vi "Control Panel.vi"(8 "error in (no error)":errorcluster, 11 "Magna Power in":refnum<class "Magna Power.lvclass">) -> (0 "error out":errorcluster, 3 "Magna Power out":refnum<class "Magna Power.lvclass">)   [LabVIEW 2017, in "Magna Power.lvclass"]
doc: "(Dynamic) A user-level application that simulates the physical front panel of the Instrument. Provide the user with buttons to manually control features of the instrument, and provide indicators of its current state."
uses:
  Magna Power.lvclass
  Magna Power.lvclass/Magna Power.ctl
panel:
  in  "Reset Power Supply":bool
  in  "Zero field":bool
  out "Actual Voltage (V)":dbl
  out "Actual Current (A)":dbl format="%.3f"
  out "Positive?":bool
  out "Status":string
  out "Field (T)":dbl format="%_4g"
  in  "Specify\nCurrent or Field?":bool=TRUE
  in  "Desired Field":dbl format="%.3f"
  in  "Read":bool
  in  "Send to power supply":bool
  in  "stop":bool
  in  "Voltage Limit":dbl=2255.0 format="%.2f"
  in  "Desired Current":dbl format="%.3f"
  in  "On?":bool
  in  "Read Continuously?":bool=TRUE
  in  "Time between reads (ms)":i32
  # "Note: Current/voltage may take 2-3 sec to update\nafter the supply is turned on."
  # "Read from Power Supply"
  # "Power Supply Control"
  # "Max ~ 1.37 T\n(Always positive,\nwill coerce > 1.37)"
  # "Max = 2255 V"
  # "Max ~ 2.184 A"
  # "Magnetic Field"
  # "(Right to left?)"
  # "A positive field corresponds to a north pole located\non the right when looking straight on at magnet"
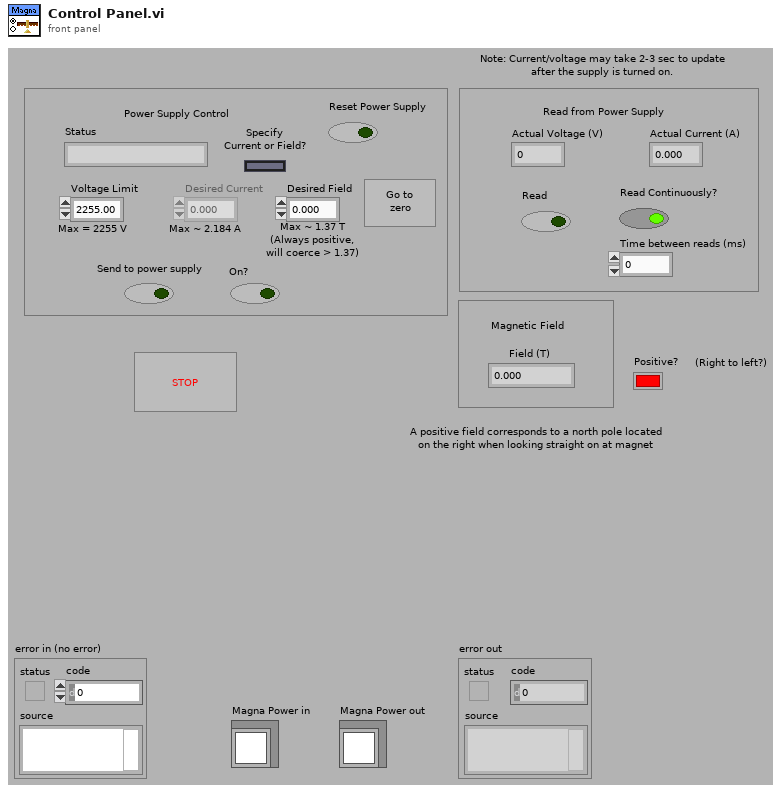
[diagram p1: front panel]
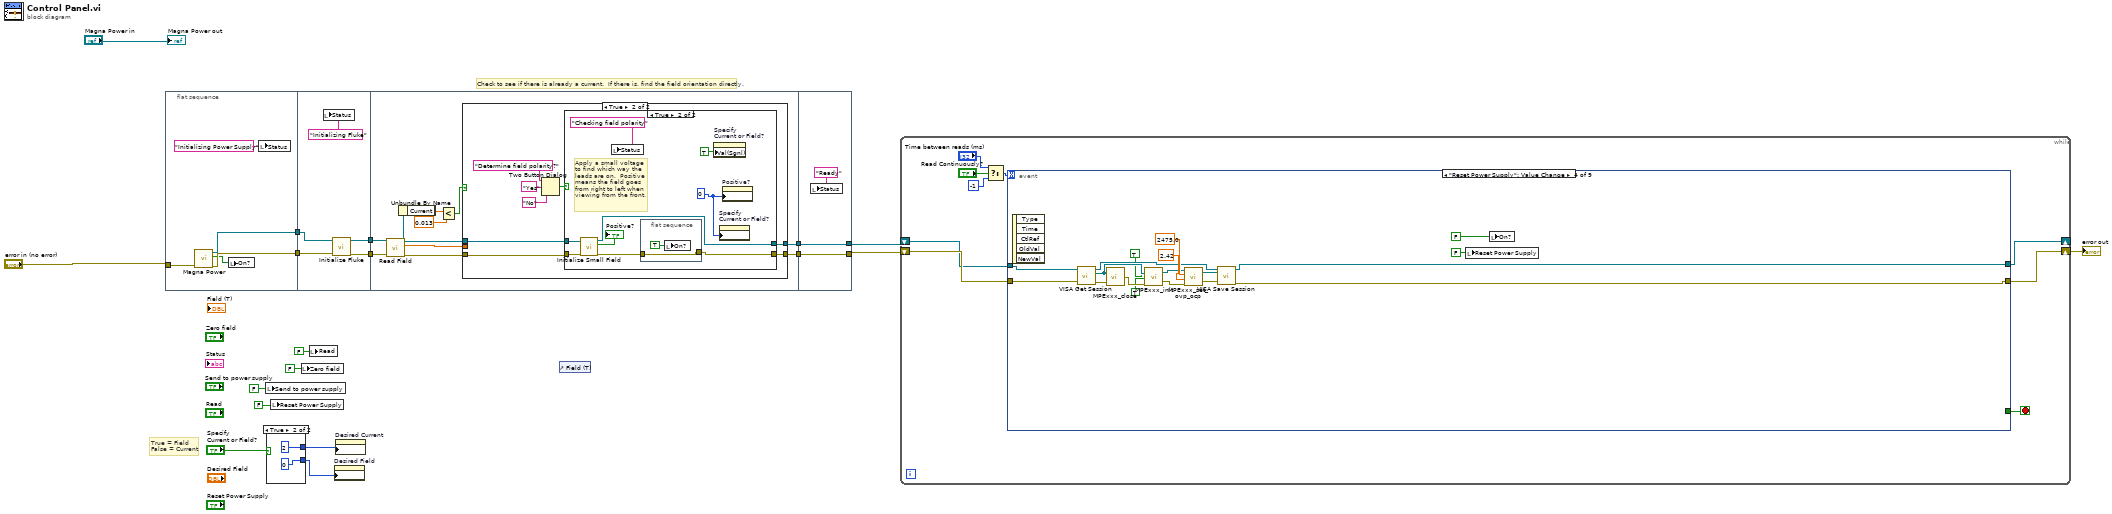
[diagram p0: block diagram]
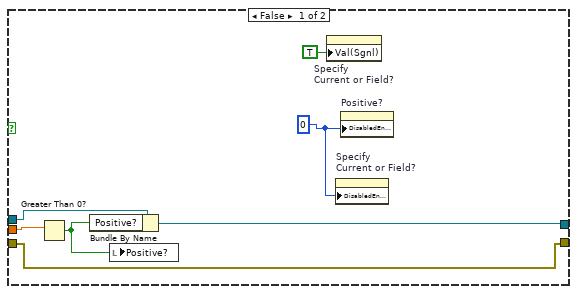
[diagram p2: hidden frame]
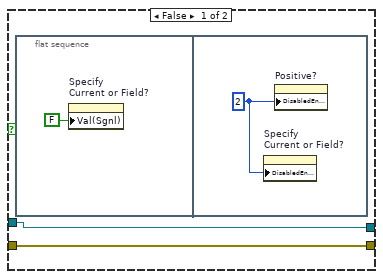
[diagram p3: hidden frame]
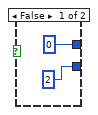
[diagram p4: hidden frame]
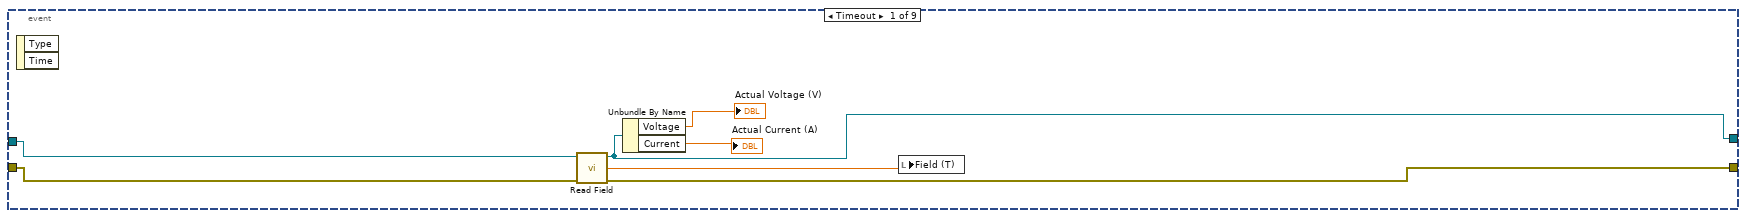
[diagram p5: hidden frame]
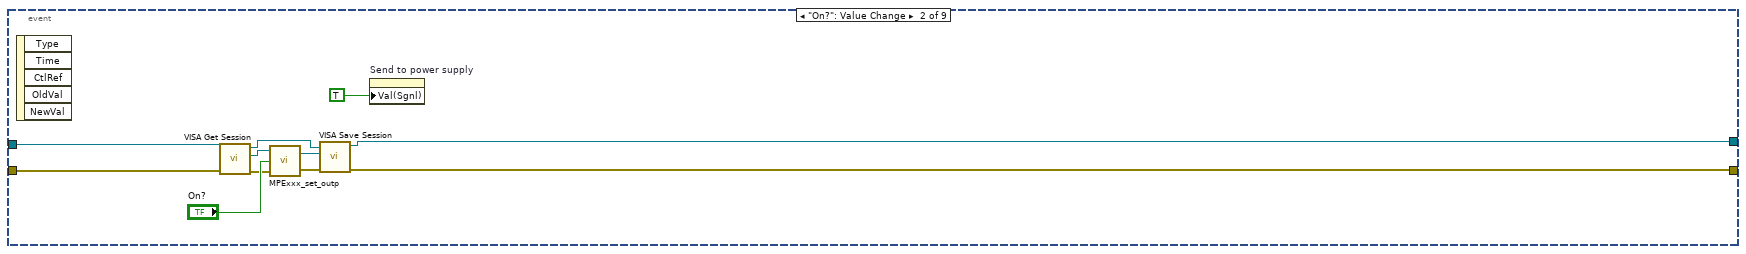
[diagram p6: hidden frame]
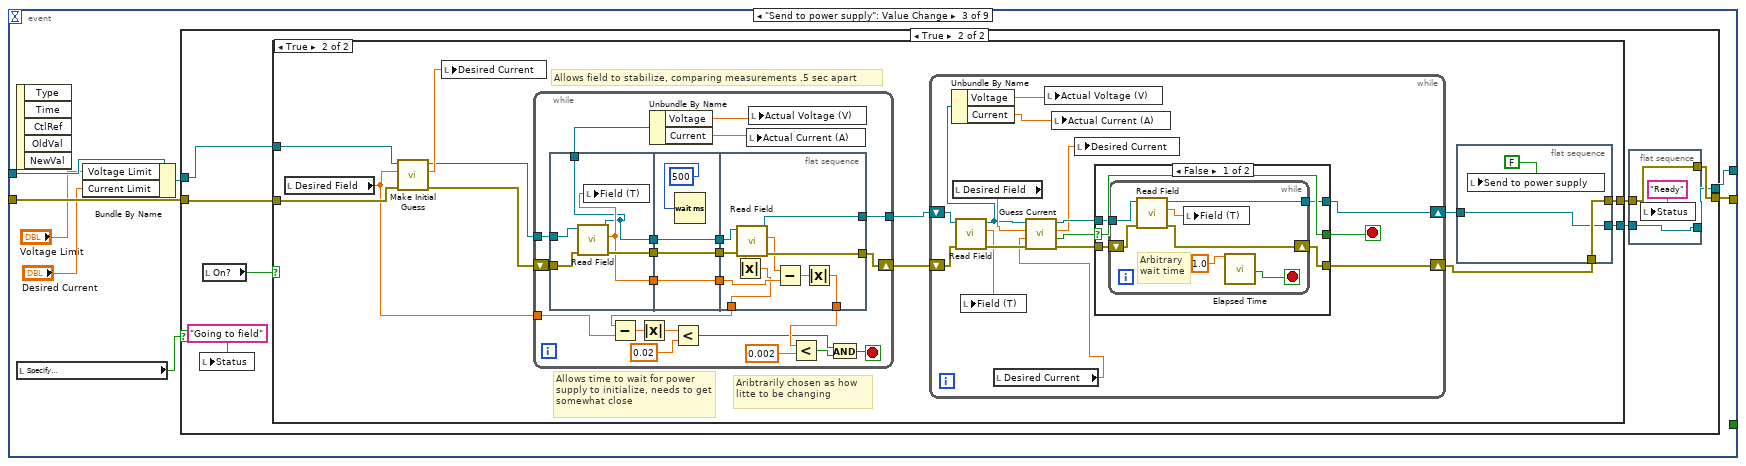
[diagram p7: hidden frame]
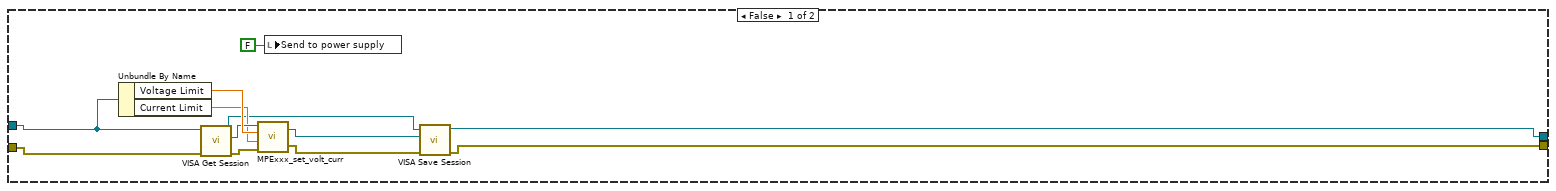
[diagram p8: hidden frame]
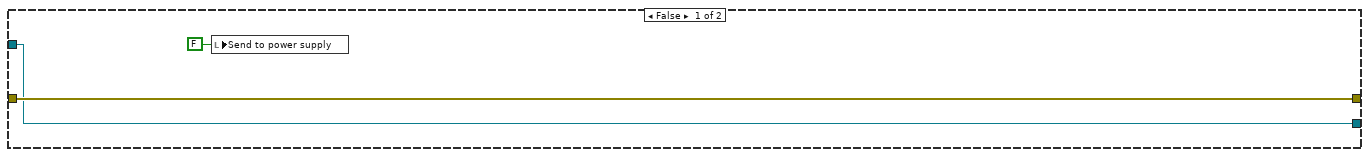
[diagram p9: hidden frame]
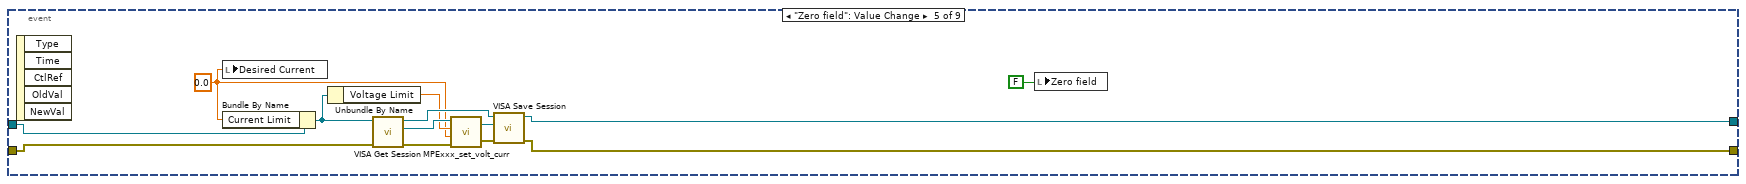
[diagram p11: hidden frame]
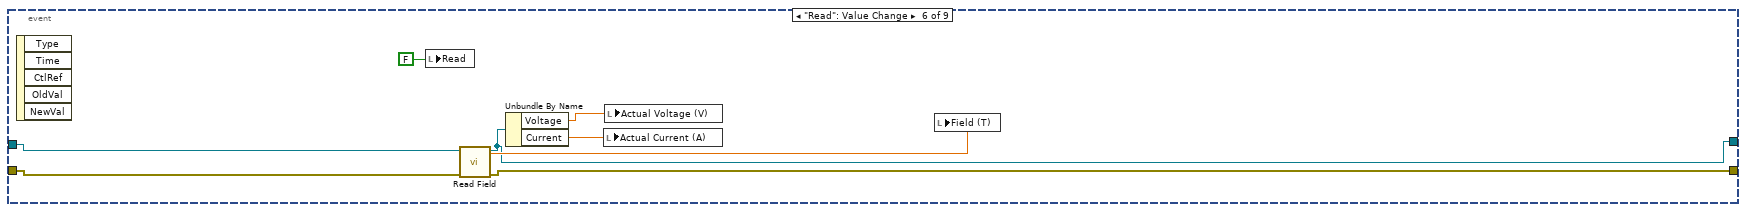
[diagram p12: hidden frame]
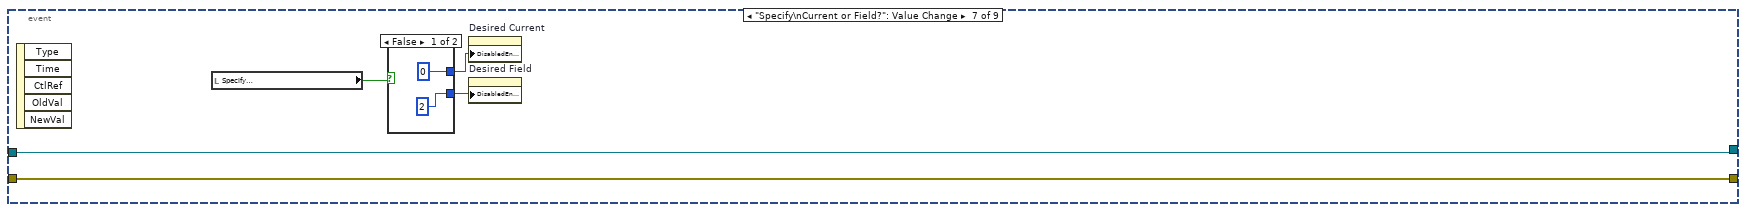
[diagram p13: hidden frame]
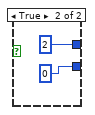
[diagram p14: hidden frame]
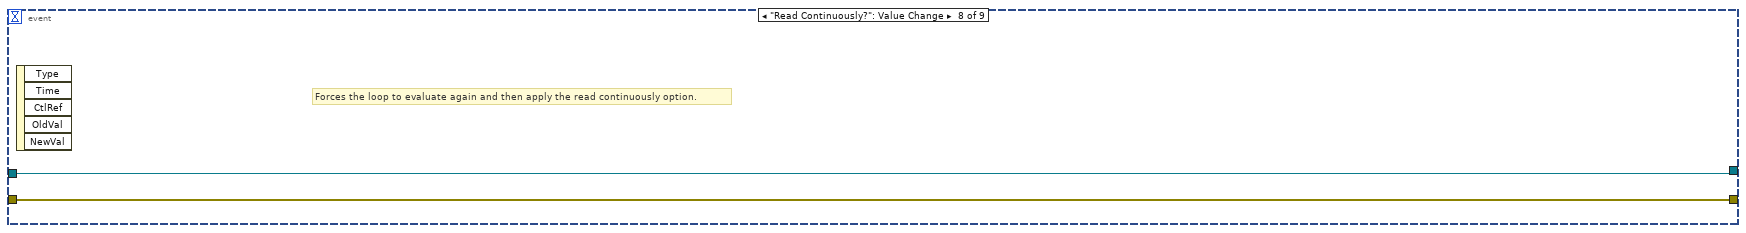
[diagram p15: hidden frame]
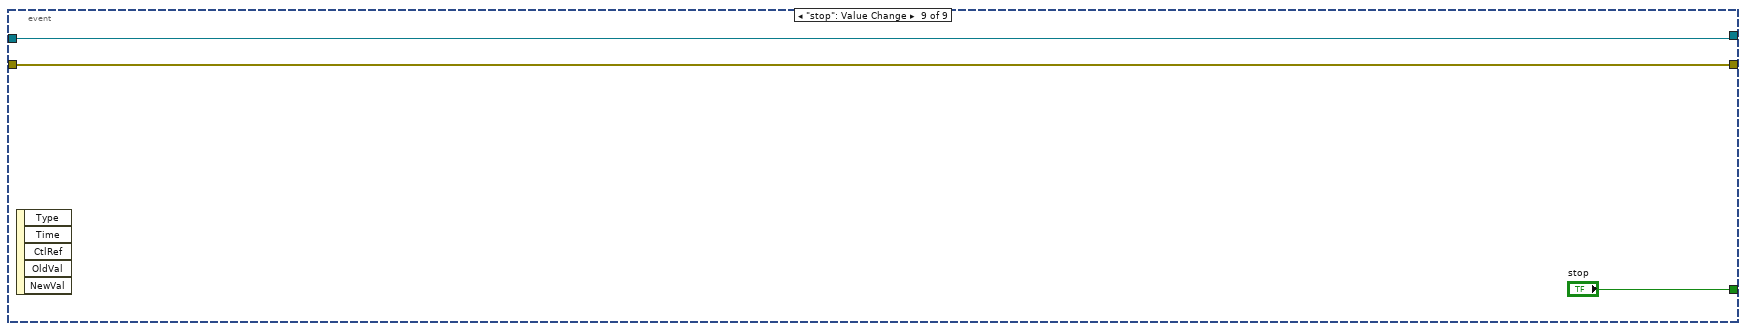
[diagram p16: hidden frame]
diagram:
  # "Check to see if there is already a current.  If there is, find the field orientation directly."
  # "True = Field\nFalse = Current"
  n1 = flat-sequence {
    tunnel: "error in (no error)" -> [w22]
    tunnel: [w21] -> w17
    tunnel: [w20] -> w7
    tunnel: w17 -> [w24]
    tunnel: [w27] -> w16
    tunnel: w7 -> [w25]
    tunnel: [w26] -> w1
    tunnel: w16 -> [w36]
    tunnel: [w38] -> w15
    tunnel: [w37] -> w14
    tunnel: w1 -> [w29]
    tunnel: [w70] -> w9
    tunnel: [w71] -> w10
    tunnel: w15 -> [w71]
    tunnel: w14 -> [w70]
    frame #0 {
      n2 = call "Magna Power.vi"("error in (no error)"=w22) -> ("error out"=w21:errorcluster, "On?"=w19:bool, "Magna Power out"=w20:refnum<class "Magna Power.lvclass">)  [unwired: 8 in]
      n3 = local write "On?"(w19) -> ()
      n4 = local write "Status"("Initializing Power Supply" ("Status")) -> ()
    }
    frame #1 {
      n5 = local write "Status"("Initializing Fluke" ("Status")) -> ()
      n6 = call "Initialize Fluke.vi"("error in (no error)"=w24, "Magna Power in"=w25) -> ("error out"=w27:errorcluster, "Magna Power out"=w26:refnum<class "Magna Power.lvclass">)  [unwired: 8 in]
    }
    frame #2 {
      n7 = call "Read Field.vi"("error in (no error)"=w36, "Magna Power in"=w29) -> ("error out"=w32:errorcluster, "Field (T)"=w30:dbl, "Magna Power out"=w31:refnum<class "Magna Power.lvclass">)  [unwired: 5 in, 2 out]
      n8 = Unbundle By Name(w31) -> ("Current"=w35:dbl)
      n9 = Less?(x=w35, y=0.013) -> (x < y?=w33:bool)
      n10 = case shown="True" w33 {
        tunnel: [w42 w53] -> w38
        tunnel: [w41 w52] -> w37
        tunnel: w32 -> [w41 w47]
        tunnel: w31 -> [w44 w46]
        tunnel: w30 -> [w45 _]
        frame False {
          w40 = 0
          n11 = Greater Than 0?(x=w45) -> (x > 0?=w43:bool)
          n12 = Bundle By Name(cluster=w44, "Positive?"=w43) -> (w42:refnum<class "Magna Power.lvclass">)
          n13 = local write "Positive?"(w43) -> ()
          n14 = property on="Specify\nCurrent or Field?" class="Bool (strict)"("Val(Sgnl)"=TRUE ("Value (Signaling)")) -> ()  [unwired: 2 in, 2 out]
          n15 = property on="Specify\nCurrent or Field?" class="Bool (strict)"("DisabledEnum"=w40) -> ()  [unwired: 2 in, 2 out]
          n16 = property on="Positive?" class="Bool (strict)"("DisabledEnum"=w40) -> ()  [unwired: 2 in, 2 out]
        }
        frame True {
          n17 = Two Button Dialog(message="Determine field polarity?", 1:"No" ("F button name (\"Cancel\")"), 2:"Yes" ("T button name (\"OK\")")) -> (T button?=w51:bool)
          n18 = case shown="True" w51 {
            tunnel: [w54 w60] -> w53
            tunnel: [w55 w58] -> w52
            tunnel: w47 -> [w55 w66]
            tunnel: w46 -> [w54 w61]
            frame False {
              n19 = flat-sequence {
                frame #0 {
                  n20 = property on="Specify\nCurrent or Field?" class="Bool (strict)"("Val(Sgnl)"=FALSE ("Value (Signaling)")) -> ()  [unwired: 2 in, 2 out]
                }
                frame #1 {
                  w57 = 2
                  n21 = property on="Specify\nCurrent or Field?" class="Bool (strict)"("DisabledEnum"=w57) -> ()  [unwired: 2 in, 2 out]
                  n22 = property on="Positive?" class="Bool (strict)"("DisabledEnum"=w57) -> ()  [unwired: 2 in, 2 out]
                }
              }
            }
            frame True {
              w63 = 0
              # "Apply a small voltage\nto find which way the\nleads are on.  Positive\nmeans the field goes\nfrom right to left when\nviewing from the front."
              n23 = call "Initialize Small Field.vi"("error in (no error)"=w66, "Magna Power in"=w61) -> ("error out"=w59:errorcluster, "Positive?"=→"Positive?":bool, "Magna Power out"=w60:refnum<class "Magna Power.lvclass">)  [unwired: 7 in]
              n24 = local write "Status"("Checking field polarity" ("Status")) -> ()
              n25 = flat-sequence {
                tunnel: w59 -> [w67]
                tunnel: [w67] -> w58
                frame #0 {
                  n26 = local write "On?"(TRUE ("On?")) -> ()
                }
              }
              n27 = property on="Specify\nCurrent or Field?" class="Bool (strict)"("Val(Sgnl)"=TRUE ("Value (Signaling)")) -> ()  [unwired: 2 in, 2 out]
              n28 = property on="Specify\nCurrent or Field?" class="Bool (strict)"("DisabledEnum"=w63) -> ()  [unwired: 2 in, 2 out]
              n29 = property on="Positive?" class="Bool (strict)"("DisabledEnum"=w63) -> ()  [unwired: 2 in, 2 out]
            }
          }
        }
      }
    }
    frame #3 {
      n30 = local write "Status"("Ready" ("Status")) -> ()
    }
  }
  n31 = local write "Send to power supply"(FALSE ("Send to power supply")) -> ()
  n32 = case shown="True" "Specify\nCurrent or Field?" {
    tunnel: [2 0] -> w11
    tunnel: [0 2] -> w12
    frame False {
    }
    frame True {
    }
  }
  n33 = local write "Reset Power Supply"(FALSE ("Send to power supply")) -> ()
  n34 = local write "Zero field"(FALSE ("Send to power supply")) -> ()
  n35 = local write "Read"(FALSE ("Send to power supply")) -> ()
  n36 = property on="Desired Field" class="DigNum (strict)"("DisabledEnum"=w11) -> ()  [unwired: 2 in, 2 out]
  n37 = property on="Desired Current" class="DigNum (strict)"("DisabledEnum"=w12) -> ()  [unwired: 2 in, 2 out]
  n38 = control-ref of="Field (T)"() -> ()  [unwired: 1 out]
  n39 = while {
    shift-right: [w78] -> w3
    shift-left: w9 -> [w80]
    shift-right: [w76] -> _
    shift-left: w10 -> [w77]
    stop <- w79 stop-if-true
    n40 = Select(t="Time between reads (ms)", s="Read Continuously?", f=-1) -> (s? t:f=w84:i32)
    n41 = event shown="[3] \"Reset Power Supply\": Value Change" {
      selector: _ -> [_ _ _ _ _ _ _ _ _]
      dyn-events: _ -> [_ _ _ _ _ _ _ _ _]
      timeout: w84 -> [_ _ _ _ _ _ _ _ _]
      tunnel: w77 -> [w90 w96 w106 w240 w253 w259 w263 w272 w274]
      tunnel: w80 -> [w89 w95 w110 w241 w252 w258 w267 w273 w275]
      tunnel: [_ _ _ _ _ _ _ _ "stop"] -> w79
      tunnel: [w88 w93 w109 w227 w243 w261 w267 w273 w275] -> w78
      tunnel: [w87 w92 w107 w228 w242 w257 w263 w272 w274] -> w76
      event Timeout {
        n42 = event-data() -> ()  [unwired: 1 in, 2 out]
        n43 = call "Read Field.vi"("error in (no error)"=w89, "Magna Power in"=w90) -> ("error out"=w88:errorcluster, "Field (T)"=w91:dbl, "Magna Power out"=w87:refnum<class "Magna Power.lvclass">)  [unwired: 5 in, 2 out]
        n44 = Unbundle By Name(w87) -> ("Voltage"=→"Actual Voltage (V)":dbl, "Current"=→"Actual Current (A)":dbl)
        n45 = local write "Field (T)"(w91) -> ()
      }
      event "On?": Value Change {
        n46 = event-data() -> ()  [unwired: 1 in, 5 out]
        n47 = call-dynamic "VISA Get Session.vi"("error in (no error)"=w95, "Instrument.lvclass in"=w96) -> ("error out"=w100:errorcluster, "VISA Resource Name"=w99:refnum<visa-resource-name>, "Instrument.lvclass out"=w94:refnum<class "Magna Power.lvclass">)  [unwired: 6 in, 1 out]
        n48 = call "MPExxx_set_outp.vi"("error in (no error)"=w100, "Output Control"="On?", "VISA session"=w99) -> ("error out"=w98:errorcluster, "dup VISA session"=w97:refnum<visa-resource-name>)
        n49 = call-dynamic "VISA Save Session.vi"("error in (no error)"=w98, "VISA Resource Name"=w97, "Instrument.lvclass in"=w94) -> ("error out"=w93:errorcluster, "Instrument.lvclass out"=w92:refnum<class "Magna Power.lvclass">)  [unwired: 7 in]
        n50 = property on="Send to power supply" class="Bool (strict)"("Val(Sgnl)"=TRUE) -> ()  [unwired: 2 in, 2 out]
      }
      event "Send to power supply": Value Change {
        n51 = event-data() -> ()  [unwired: 1 in, 5 out]
        n52 = local read "Specify\nCurrent or Field?"() -> (w108:bool)
        n53 = Bundle By Name(cluster=w106, "Voltage Limit"="Voltage Limit", "Current Limit"="Desired Current") -> (w105:refnum<class "Magna Power.lvclass">)
        n54 = case shown="True" w108 {
          tunnel: w105 -> [w111 w129]
          tunnel: w110 -> [w121 w130]
          tunnel: [w116 w126] -> w109
          tunnel: [w118 w124] -> w107
          frame False {
            n55 = Unbundle By Name(w111) -> ("Voltage Limit"=w117:dbl, "Current Limit"=w113:dbl)
            n56 = call-dynamic "VISA Get Session.vi"("error in (no error)"=w121, "Instrument.lvclass in"=w111) -> ("error out"=w120:errorcluster, "VISA Resource Name"=w115:refnum<visa-resource-name>, "Instrument.lvclass out"=w112:refnum<class "Magna Power.lvclass">)  [unwired: 6 in, 1 out]
            n57 = call "MPExxx_set_volt_curr.vi"("error in (no error)"=w120, "Set Current"=w113, "Set Voltage"=w117, "VISA session"=w115) -> ("error out"=w119:errorcluster, "dup VISA session"=w114:refnum<visa-resource-name>)
            n58 = local write "Send to power supply"(FALSE) -> ()
            n59 = call-dynamic "VISA Save Session.vi"("error in (no error)"=w119, "VISA Resource Name"=w114, "Instrument.lvclass in"=w112) -> ("error out"=w116:errorcluster, "Instrument.lvclass out"=w118:refnum<class "Magna Power.lvclass">)  [unwired: 7 in]
          }
          frame True {
            n60 = local write "Status"("Going to field" ("Status")) -> ()
            n61 = local read "On?"() -> (w128:bool)
            n62 = case shown="True" w128 {
              tunnel: w130 -> [w136 w148]
              tunnel: [w136 w144] -> w125
              tunnel: w129 -> [w134 w147]
              tunnel: [w134 w138] -> w123
              frame False {
                n63 = local write "Send to power supply"(FALSE ("Send to power supply")) -> ()
              }
              frame True {
                # "Allows field to stabilize, comparing measurements .5 sec apart"
                # "Allows time to wait for power supply to initialize, needs to get somewhat close"
                # "Aribtrarily chosen as how litte to be changing"
                n64 = local read "Desired Field"() -> (w141:dbl)
                n65 = call "Make Initial Guess.vi"("error in (no error)"=w148, "Desired Field"=w141, "Magna Power in"=w147) -> ("error out"=w139:errorcluster, "First guess"=w146:dbl, "Magna Power out"=w140:refnum<class "Magna Power.lvclass">)  [unwired: 6 in]
                n66 = local write "Desired Current"(w146) -> ()
                n67 = while {
                  shift-right: [w199] -> w145
                  shift-left: w139 -> [w205]
                  tunnel: w140 -> [w197]
                  tunnel: [w194] -> w142
                  tunnel: w141 -> [w190]
                  stop <- w193 stop-if-true
                  n68 = flat-sequence {
                    tunnel: w205 -> [w210]
                    tunnel: [w209] -> w203
                    tunnel: [w208] -> w201
                    tunnel: w197 -> [w207]
                    tunnel: [w206] -> w195
                    tunnel: [w206] -> w185
                    tunnel: [w213] -> w204
                    tunnel: w203 -> [w213]
                    tunnel: [w212] -> w202
                    tunnel: w201 -> [w212]
                    tunnel: [w211] -> w196
                    tunnel: w195 -> [w211]
                    tunnel: w204 -> [w223]
                    tunnel: w202 -> [w217]
                    tunnel: [w221] -> w198
                    tunnel: [w220] -> w199
                    tunnel: w196 -> [w218]
                    tunnel: [w219] -> w194
                    tunnel: [w215] -> w191
                    frame #0 {
                      n69 = call "Read Field.vi"("error in (no error)"=w210, "Magna Power in"=w207) -> ("error out"=w209:errorcluster, "Field (T)"=w208:dbl, "Magna Power out"=w206:refnum<class "Magna Power.lvclass">)  [unwired: 5 in, 2 out]
                      n70 = local write "Field (T)"(w208) -> ()
                    }
                    frame #1 {
                      n71 = Wait (ms)(milliseconds to wait=u32 500) -> ()  [unwired: 1 out]
                    }
                    frame #2 {
                      n72 = call "Read Field.vi"("error in (no error)"=w223, "Magna Power in"=w218) -> ("error out"=w220:errorcluster, "Field (T)"=w216:dbl, "Magna Power out"=w219:refnum<class "Magna Power.lvclass">)  [unwired: 5 in, 2 out]
                      n73 = Absolute Value(x=w216) -> (abs(x)=w215:dbl)
                      n74 = Subtract(x=w216, y=w217) -> (x-y=w222:dbl)
                      n75 = Absolute Value(x=w222) -> (abs(x)=w221:dbl)
                    }
                  }
                  n76 = Subtract(x=w191, y=w190) -> (x-y=w189:dbl)
                  n77 = Absolute Value(x=w189) -> (abs(x)=w188:dbl)
                  n78 = Unbundle By Name(w185) -> ("Voltage"=w184:dbl, "Current"=w183:dbl)
                  n79 = Less?(x=w188, y=0.02) -> (x < y?=w186:bool)
                  n80 = local write "Actual Current (A)"(w183) -> ()
                  n81 = local write "Actual Voltage (V)"(w184) -> ()
                  n82 = Less?(x=w198, y=0.002) -> (x < y?=w192:bool)
                  n83 = And(x=w186, y=w192) -> (x .and. y?=w193:bool)
                }
                n84 = while {
                  shift-right: [w163] -> w143
                  shift-left: w145 -> [w167]
                  shift-right: [w154] -> w137
                  shift-left: w142 -> [w162]
                  stop <- w156 stop-if-true
                  n85 = local read "Desired Field"() -> (w159:dbl)
                  n86 = call "Read Field.vi"("error in (no error)"=w167, "Magna Power in"=w162) -> ("error out"=w166:errorcluster, "Field (T)"=w158:dbl, "Magna Power out"=w155:refnum<class "Magna Power.lvclass">)  [unwired: 5 in, 2 out]
                  n87 = Unbundle By Name(w155) -> ("Voltage"=w153:dbl, "Current"=w152:dbl)
                  n88 = local write "Field (T)"(w158) -> ()
                  n89 = local read "Desired Current"() -> (w157:dbl)
                  n90 = call "Guess Current.vi"("error in (no error)"=w166, "Current guess"=w157, "Desired Field"=w159, "Magna Power in"=w155) -> ("error out"=w164:errorcluster, "Stop?"=w165:bool, "New guess"=w160:dbl, "Magna Power out"=w161:refnum<class "Magna Power.lvclass">)  [unwired: 4 in]
                  n91 = local write "Actual Voltage (V)"(w153) -> ()
                  n92 = local write "Actual Current (A)"(w152) -> ()
                  n93 = local write "Desired Current"(w160) -> ()
                  n94 = case shown="False" w165 {
                    selector: w165 -> [w171 w182]
                    tunnel: [w171 w182] -> w156
                    tunnel: w164 -> [w172 w181]
                    tunnel: [w170 w181] -> w163
                    tunnel: w161 -> [w169 w180]
                    tunnel: [w168 w180] -> w154
                    frame False {
                      n95 = while {
                        shift-right: [w177] -> w170
                        shift-left: w172 -> [w179]
                        tunnel: w169 -> [w175]
                        tunnel: [w173] -> w168
                        stop <- w174 stop-if-true
                        # "Arbitrary\nwait time"
                        n96 = call "Read Field.vi"("error in (no error)"=w179, "Magna Power in"=w175) -> ("error out"=w177:errorcluster, "Field (T)"=w178:dbl, "Magna Power out"=w173:refnum<class "Magna Power.lvclass">)  [unwired: 5 in, 2 out]
                        n97 = local write "Field (T)"(w178) -> ()
                        n98 = call "Elapsed Time"("Time Target (s)"=1.0) -> ("Time has Elapsed"=w174:bool)  [unwired: 11 in, 7 out]
                      }
                    }
                    frame True {
                    }
                  }
                }
                n99 = flat-sequence {
                  tunnel: [w150] -> w144
                  tunnel: w143 -> [w150]
                  tunnel: [w149] -> w138
                  tunnel: w137 -> [w149]
                  frame #0 {
                    n100 = local write "Send to power supply"(FALSE) -> ()
                  }
                }
              }
            }
            n101 = flat-sequence {
              tunnel: [w132] -> w126
              tunnel: w125 -> [w132]
              tunnel: [w131] -> w124
              tunnel: w123 -> [w131]
              frame #0 {
                n102 = local write "Status"("Ready" ("Status")) -> ()
              }
            }
          }
        }
      }
      event "Reset Power Supply": Value Change {
        n103 = event-data() -> ()  [unwired: 1 in, 5 out]
        n104 = call-dynamic "VISA Get Session.vi"("error in (no error)"=w241, "Instrument.lvclass in"=w240) -> ("error out"=w239:errorcluster, "VISA Resource Name"=w237:refnum<visa-resource-name>, "Instrument.lvclass out"=w230:refnum<class "Magna Power.lvclass">)  [unwired: 6 in, 1 out]
        n105 = call "MPExxx_close.vi"("error in (no error)"=w239, "VISA session"=w237) -> ("error out"=w238:errorcluster)
        n106 = call "MPExxx_init.vi"("error in (no error)"=w238, "ID Query (T: Query)"=TRUE ("Reset Device (T: Reset)"), "Reset Device (T: Reset)"=TRUE ("ID Query (T: Query)"), "VISA session"=w237) -> ("error out"=w234:errorcluster, "dup VISA session"=w233:refnum<visa-resource-name>)
        n107 = call "MPExxx_set_ovp_ocp.vi"("error in (no error)"=w234, "Set OCP"=2.42 ("OCP"), "Set OVP"=2475.0 ("OVP"), "VISA session"=w233) -> ("error out"=w231:errorcluster, "dup VISA session"=w232:refnum<visa-resource-name>)
        n108 = call-dynamic "VISA Save Session.vi"("error in (no error)"=w231, "VISA Resource Name"=w232, "Instrument.lvclass in"=w230) -> ("error out"=w227:errorcluster, "Instrument.lvclass out"=w228:refnum<class "Magna Power.lvclass">)  [unwired: 7 in]
        n109 = local write "Reset Power Supply"(FALSE ("Reset Power Supply")) -> ()
        n110 = local write "On?"(FALSE ("Reset Power Supply")) -> ()
      }
      event "Zero field": Value Change {
        w244 = 0.0 ("Desired Current")
        n111 = event-data() -> ()  [unwired: 1 in, 5 out]
        n112 = local write "Desired Current"(w244) -> ()
        n113 = Bundle By Name(cluster=w253, "Current Limit"=w244) -> (w246:refnum<class "Magna Power.lvclass">)
        n114 = Unbundle By Name(w246) -> ("Voltage Limit"=w245:dbl)
        n115 = call-dynamic "VISA Get Session.vi"("error in (no error)"=w252, "Instrument.lvclass in"=w246) -> ("error out"=w251:errorcluster, "VISA Resource Name"=w247:refnum<visa-resource-name>, "Instrument.lvclass out"=w248:refnum<class "Magna Power.lvclass">)  [unwired: 6 in, 1 out]
        n116 = call "MPExxx_set_volt_curr.vi"("error in (no error)"=w251, "Set Current"=w244, "Set Voltage"=w245, "VISA session"=w247) -> ("error out"=w250:errorcluster, "dup VISA session"=w249:refnum<visa-resource-name>)
        n117 = call-dynamic "VISA Save Session.vi"("error in (no error)"=w250, "VISA Resource Name"=w249, "Instrument.lvclass in"=w248) -> ("error out"=w243:errorcluster, "Instrument.lvclass out"=w242:refnum<class "Magna Power.lvclass">)  [unwired: 7 in]
        n118 = local write "Zero field"(FALSE ("Send to power supply")) -> ()
      }
      event "Read": Value Change {
        n119 = event-data() -> ()  [unwired: 1 in, 5 out]
        n120 = local write "Read"(FALSE) -> ()
        n121 = call "Read Field.vi"("error in (no error)"=w258, "Magna Power in"=w259) -> ("error out"=w261:errorcluster, "Field (T)"=w260:dbl, "Magna Power out"=w257:refnum<class "Magna Power.lvclass">)  [unwired: 5 in, 2 out]
        n122 = Unbundle By Name(w257) -> ("Voltage"=w256:dbl, "Current"=w255:dbl)
        n123 = local write "Actual Current (A)"(w255) -> ()
        n124 = local write "Actual Voltage (V)"(w256) -> ()
        n125 = local write "Field (T)"(w260) -> ()
      }
      event "Specify\nCurrent or Field?": Value Change {
        n126 = event-data() -> ()  [unwired: 1 in, 5 out]
        n127 = local read "Specify\nCurrent or Field?"() -> (w266:bool)
        n128 = case shown="False" w266 {
          tunnel: [2 0] -> w265
          tunnel: [0 2] -> w264
          frame False {
          }
          frame True {
          }
        }
        n129 = property on="Desired Current" class="DigNum (strict)"("DisabledEnum"=w264) -> ()  [unwired: 2 in, 2 out]
        n130 = property on="Desired Field" class="DigNum (strict)"("DisabledEnum"=w265) -> ()  [unwired: 2 in, 2 out]
      }
      event "Read Continuously?": Value Change {
        # "Forces the loop to evaluate again and then apply the read continuously option."
        n131 = event-data() -> ()  [unwired: 1 in, 5 out]
      }
      event "stop": Value Change {
        n132 = event-data() -> ()  [unwired: 1 in, 5 out]
      }
    }
  }
  "error out" <- w3
  "Magna Power out" <- "Magna Power in"
